vi "get name of mapped tag from channel.vi"(8 "error in (no error)":errorcluster, 9 "channel":refnum<class "TBM channel.lvclass">, 10 "engine in":refnum<class "Engine Parent Editor Node.lvclass">, 11 "editor node in":refnum<class "module editor node.lvclass">) -> (0 "error out":errorcluster, 1 "tag name":string, 2 "engine out":refnum<class "Engine Parent Editor Node.lvclass">, 3 "editor node out":refnum<class "module editor node.lvclass">)   [LabVIEW 2013, in "Shared Memory editor node.lvclass"]
uses:
  Shared Memory editor node.lvclass
  <vilib>/NI/DCAF/Tag Editor Core/Configuration Editor/Classes/Module editor node/module editor node.lvclass
  <vilib>/NI/DCAF/Tag Editor Core/Configuration Editor/Classes/Engine Parent/Engine Parent Editor Node.lvclass
  <vilib>/NI/Tag Bus Module Framework/channel/TBM channel.lvclass
  <vilib>/NI/Configuration Framework/serializable configuration/NISE_CEF_serializable configuration.lvclass/NISE_CEF_serializable configuration.ctl
  <vilib>/NI/Tag Bus/tag/tag descriptor.lvclass/tag descriptor.ctl
  <vilib>/Utility/LVClass/Get LV Class Name.vi
  <vilib>/NI/Configuration Framework/error generator/NISE_error generator.vi
  <vilib>/NI/Module Execution Interface/Engine Configuration/engine configuration.lvclass
  <vilib>/NI/Configuration Framework/serializable configuration/NISE_CEF_serializable configuration.lvclass
  <vilib>/NI/Tag Bus/tag/tag descriptor.lvclass
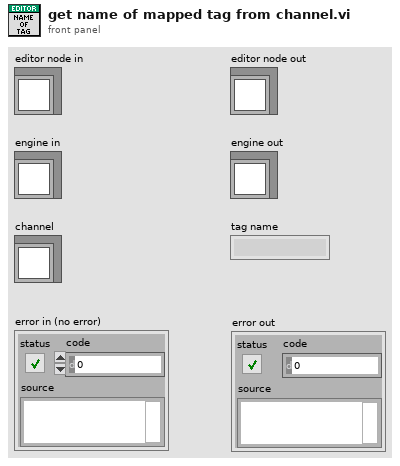
[diagram p1: front panel]
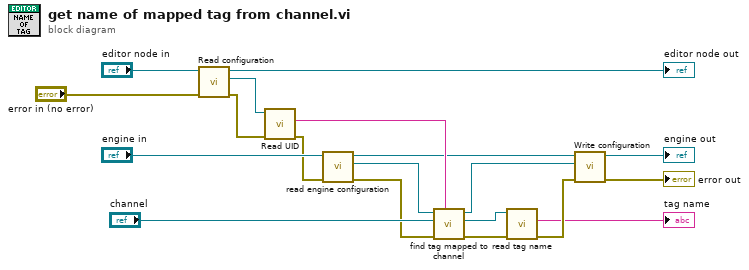
[diagram p0: block diagram]
diagram:
  n1 = call-dynamic "Read configuration.vi"("error in"="error in (no error)", "NISE_CEF_serializable node in"="editor node in") -> ("error out"=w1:errorcluster, "configuration"=w10:refnum<class "NISE_CEF_serializable configuration.lvclass">, "NISE_CEF_serializable node out"=→"editor node out":refnum<class "module editor node.lvclass">)  [unwired: 7 in]
  n2 = call <vilib>:"Read UID.vi"("error in"=w1, "configuration in"=w10) -> ("error out"=w5:errorcluster, "instance id"=w7:string)  [unwired: 7 in, 1 out]
  n3 = call <vilib>:"read engine configuration.vi"("error in"=w5, "Engine Parent Editor Node in"="engine in") -> ("error out"=w6:errorcluster, "engine configuration"=w2:refnum<class "engine configuration.lvclass">, "Engine Parent Editor Node out"=w3:refnum<class "Engine Parent Editor Node.lvclass">)  [unwired: 7 in]
  n4 = call <vilib>:"find tag mapped to channel.vi"("owner"=w7, "error in"=w6, "channel"="channel", "engine configuration in"=w2) -> ("error out"=w12:errorcluster, "tag"=w13:refnum<class "tag descriptor.lvclass">, "engine configuration out"=w4:refnum<class "engine configuration.lvclass">)  [unwired: 5 in]
  n5 = call <vilib>:"read tag name.vi"("error in"=w12, "system tag in"=w13) -> ("error out"=w15:errorcluster, "name"=→"tag name":string)  [unwired: 7 in, 1 out]
  n6 = call-dynamic "Write configuration.vi"("error in"=w15, "configuration"=w4, "NISE_CEF_serializable node in"=w3) -> ("error out"=→"error out":errorcluster, "NISE_CEF_serializable node out"=→"engine out":refnum<class "Engine Parent Editor Node.lvclass">)  [unwired: 7 in]
